vi "fpQuantizeFloat.vi"   [LabVIEW 2011]
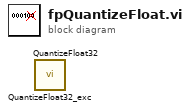
[diagram p0: block diagram]
diagram:
  n1 = call "QuantizeFloat32_exc.vi"() -> ()  [unwired: 8 in, 3 out]
  n2 = call "QuantizeFloat32.vi"() -> ()  [unwired: 10 in, 1 out]
